vi "mMc emulator.vi"(2 "Command":string, 3 "error in (no error)":errorcluster) -> (7 "Return":string, 9 "error out":errorcluster)   [LabVIEW 2013]
uses:
  mMc param - global.vi
panel:
  out "Querry?":bool
  out "Param nn":dbl format="%.2f"
  out "Cmd":string
  out "Param xx":string
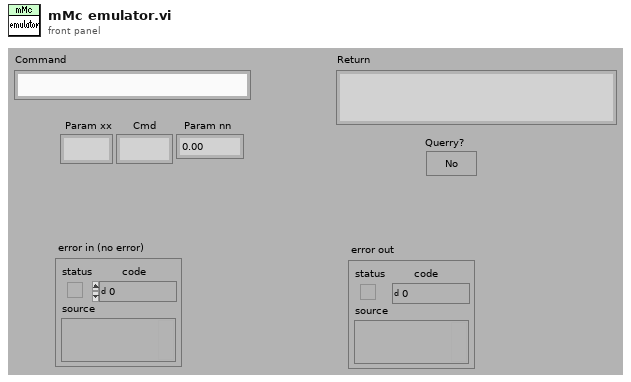
[diagram p1: front panel]
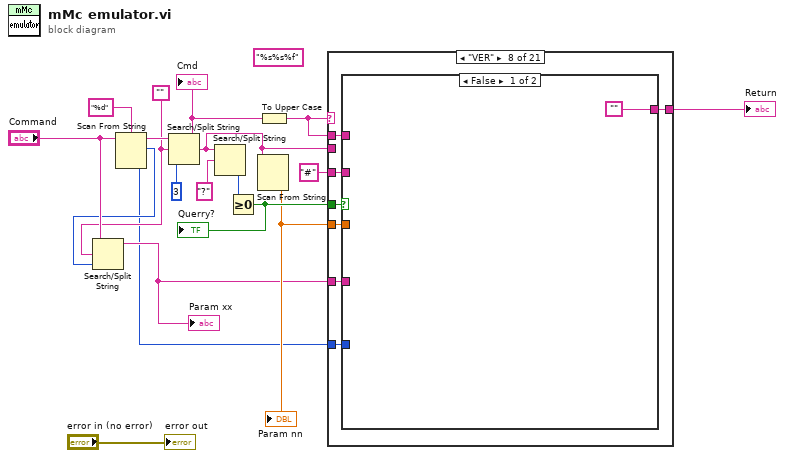
[diagram p0: block diagram]
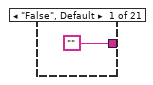
[diagram p2: hidden frame]
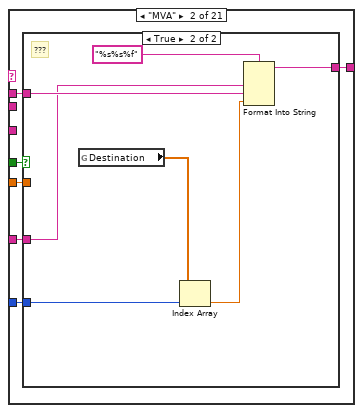
[diagram p3: hidden frame]
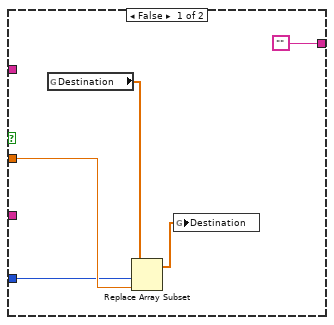
[diagram p4: hidden frame]
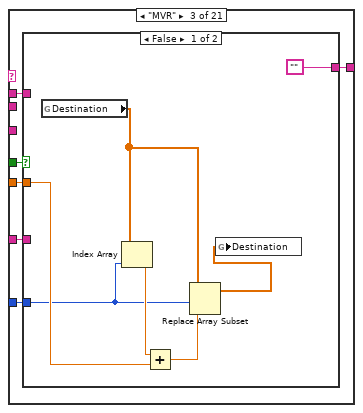
[diagram p5: hidden frame]
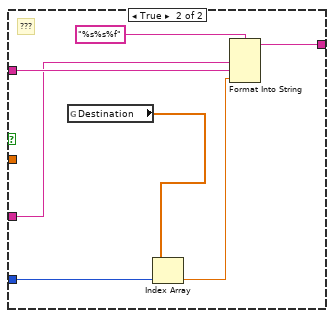
[diagram p6: hidden frame]
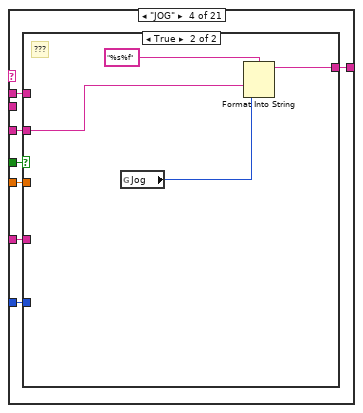
[diagram p7: hidden frame]
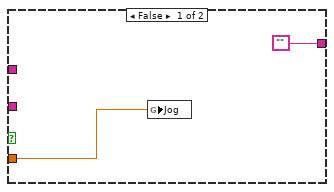
[diagram p8: hidden frame]
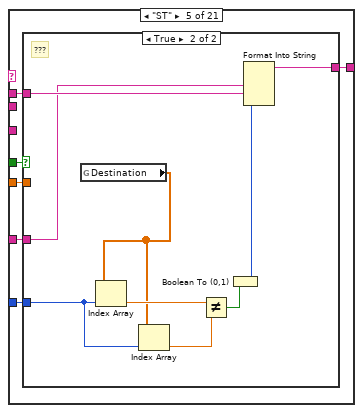
[diagram p9: hidden frame]
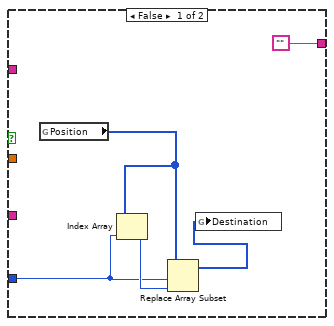
[diagram p10: hidden frame]
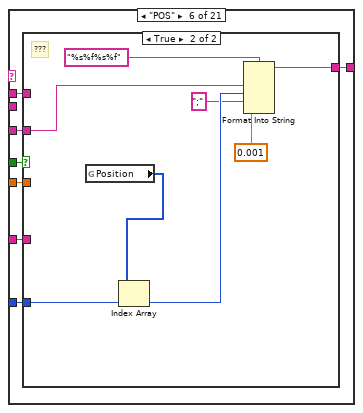
[diagram p11: hidden frame]
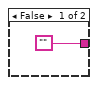
[diagram p12: hidden frame]
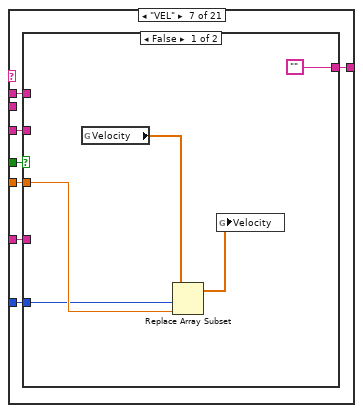
[diagram p13: hidden frame]
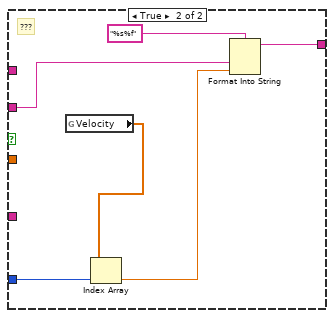
[diagram p14: hidden frame]
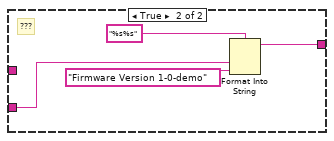
[diagram p15: hidden frame]
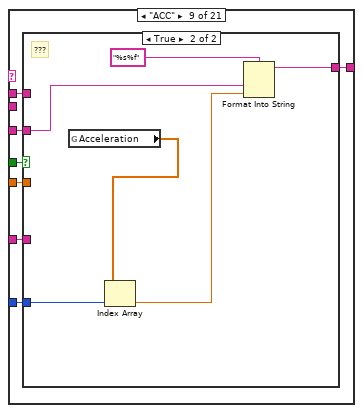
[diagram p16: hidden frame]
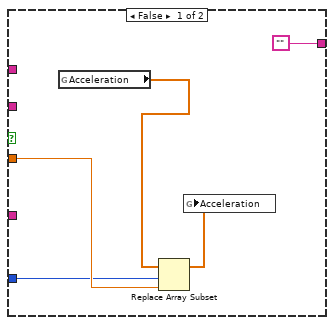
[diagram p17: hidden frame]
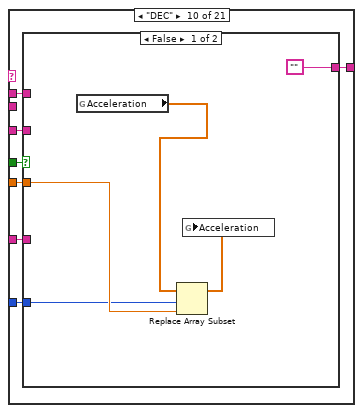
[diagram p18: hidden frame]
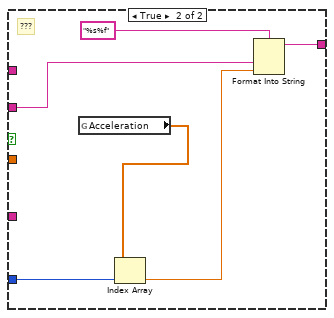
[diagram p19: hidden frame]
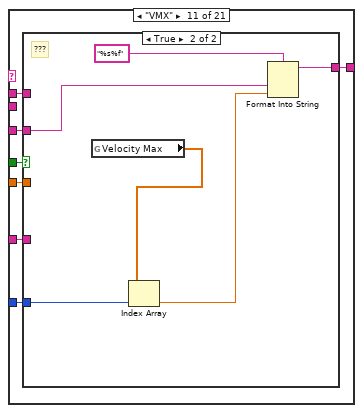
[diagram p20: hidden frame]
diagram:
  (unwired) "%s%s%f" ("Format String")
  w11 = ""
  n1 = Scan From String(format string="%d" ("Format String"), input string="Command") -> (remaining string=w18:string, offset past scan=w5:u32, output 1=w4:i32)  [unwired: 3 in, 1 out]
  n2 = Search/Split String(string="Command", search string/char (-)=w11, offset (0)=w5) -> (substring before match=w7:string)  [unwired: 2 out]
  "Param xx" <- w7
  n3 = Search/Split String(string=w18, search string/char (-)=w11, offset (0)=3) -> (substring before match=w14:string, match + rest of string=w2:string)  [unwired: 1 out]
  "Cmd" <- w14
  n4 = Search/Split String(string=w2, search string/char (-)="?") -> (offset of match=w15:i32)  [unwired: 1 in, 2 out]
  n5 = Greater Or Equal To 0?(x=w15) -> (x >= 0?=w13:bool)
  "Querry?" <- w13
  n6 = Scan From String(input string=w2) -> (output 1=w8:dbl)  [unwired: 4 in, 3 out]
  "Param nn" <- w8
  n7 = To Upper Case(1:w14) -> (0:w10:string)
  n8 = case shown="\"VER\"" w10 {
    tunnel: w13 -> [_ w25 w43 w64 w76 w97 w113 w131 w143 w161 w179 w197 w215 w233 w251 w269 w287 w305 w324 w342 w362]
    tunnel: w4 -> [_ w24 w42 w63 w75 w96 w112 w130 w142 w160 w178 w196 w214 w232 w250 w268 w286 w304 w323 w341 w361]
    tunnel: w7 -> [_ w22 w40 w61 w73 w94 w110 w128 w140 w158 w176 w194 w212 w230 w248 w266 w284 w302 w321 w339 w359]
    tunnel: w10 -> [_ w23 w41 w62 w74 w95 w111 w129 w141 w159 w177 w195 w213 w231 w249 w267 w285 w303 w322 w340 w360]
    tunnel: ["" w21 w39 w60 w72 w93 w109 w127 w139 w157 w175 w193 w211 w229 w247 w265 w283 w301 w320 w338 w358] -> w9
    tunnel: w8 -> [_ w20 w38 w59 w71 w92 w108 w126 w138 w156 w174 w192 w210 w228 w246 w264 w282 w300 w319 w337 w357]
    tunnel: w2 -> [_ _ _ _ _ _ _ _ _ _ _ _ _ _ _ _ _ _ w317 _ w356]
    tunnel: "#" ("Format String") -> [_ _ _ w58 _ w91 w107 w125 w137 w155 w173 w191 w209 w227 w245 w263 w281 w299 w318 w336 _]
    frame "False", Default {
    }
    frame "MVA" {
      n9 = case shown="True" w25 {
        tunnel: w24 -> [w26 w31]
        tunnel: w23 -> [_ w37]
        tunnel: w22 -> [_ w35]
        tunnel: ["" w34] -> w21
        tunnel: w20 -> [w29 _]
        frame False {
          n10 = global read "mMc param - global.vi" "Destination"() -> (w28:dbl[])
          n11 = Replace Array Subset(array=w28, new element=w29, index=w26) -> (w27:dbl[])
          n12 = global write "mMc param - global.vi" "Destination"(w27) -> ()
        }
        frame True {
          # "???"
          n13 = global read "mMc param - global.vi" "Destination"() -> (w32:dbl[])
          n14 = Index Array(array=w32, index=w31) -> (element=w36:dbl)
          n15 = Format Into String(format string="%s%s%f" ("Format String"), w35, w37, w36) -> (resulting string=w34:string)  [unwired: 2 in, 1 out]
        }
      }
    }
    frame "MVR" {
      n16 = case shown="False" w43 {
        tunnel: w42 -> [w44 w51]
        tunnel: w41 -> [_ w57]
        tunnel: w40 -> [_ w55]
        tunnel: ["" w54] -> w39
        tunnel: w38 -> [w49 _]
        frame False {
          n17 = global read "mMc param - global.vi" "Destination"() -> (w46:dbl[])
          n18 = Index Array(array=w46, index=w44) -> (element=w48:dbl)
          n19 = Add(x=w48, y=w49) -> (x+y=w47:dbl)
          n20 = Replace Array Subset(array=w46, new element=w47, index=w44) -> (w45:dbl[])
          n21 = global write "mMc param - global.vi" "Destination"(w45) -> ()
        }
        frame True {
          # "???"
          n22 = global read "mMc param - global.vi" "Destination"() -> (w52:dbl[])
          n23 = Index Array(array=w52, index=w51) -> (element=w56:dbl)
          n24 = Format Into String(format string="%s%s%f" ("Format String"), w55, w57, w56) -> (resulting string=w54:string)  [unwired: 2 in, 1 out]
        }
      }
    }
    frame "JOG" {
      n25 = case shown="True" w64 {
        tunnel: w63 -> [_ _]
        tunnel: w62 -> [_ _]
        tunnel: w61 -> [_ _]
        tunnel: ["" w70] -> w60
        tunnel: w59 -> [w65 _]
        tunnel: w58 -> [_ w67]
        frame False {
          n26 = global write "mMc param - global.vi" "Jog"(w65) -> ()
        }
        frame True {
          # "???"
          n27 = global read "mMc param - global.vi" "Jog"() -> (w68:i32)
          n28 = Format Into String(format string="%s%f" ("Format String"), w67, w68) -> (resulting string=w70:string)  [unwired: 2 in, 1 out]
        }
      }
    }
    frame "ST" {
      n29 = case shown="True" w76 {
        tunnel: w75 -> [w77 w82]
        tunnel: w74 -> [_ w90]
        tunnel: w73 -> [_ w89]
        tunnel: ["" w88] -> w72
        tunnel: w71 -> [_ _]
        frame False {
          n30 = global read "mMc param - global.vi" "Position"() -> (w79:i32[])
          n31 = Index Array(array=w79, index=w77) -> (element=w80:i32)
          n32 = Replace Array Subset(array=w79, new element=w80, index=w77) -> (w78:i32[])
          n33 = global write "mMc param - global.vi" "Destination"(w78) -> ()
        }
        frame True {
          # "???"
          n34 = global read "mMc param - global.vi" "Destination"() -> (w83:dbl[])
          n35 = Index Array(array=w83, index=w82) -> (element=w87:dbl)
          n36 = Index Array(array=w83, index=w82) -> (element=w86:dbl)
          n37 = Not Equal?(x=w87, y=w86) -> (x != y?=w85:bool)
          n38 = Boolean To (0,1)(Boolean=w85) -> (0, 1=w84:i16)
          n39 = Format Into String(w89, w90, w84) -> (resulting string=w88:string)  [unwired: 3 in, 1 out]
        }
      }
    }
    frame "POS" {
      n40 = case shown="True" w97 {
        tunnel: w96 -> [_ w99]
        tunnel: w95 -> [_ _]
        tunnel: w94 -> [_ _]
        tunnel: ["" w106] -> w93
        tunnel: w92 -> [_ _]
        tunnel: w91 -> [_ w102]
        frame False {
        }
        frame True {
          # "???"
          n41 = global read "mMc param - global.vi" "Position"() -> (w103:i32[])
          n42 = Index Array(array=w103, index=w99) -> (element=w105:i32)
          n43 = Format Into String(format string="%s%f%s%f" ("Format String"), w102, w105, ";" ("input 3"), 0.001 ("input 4")) -> (resulting string=w106:string)  [unwired: 2 in, 1 out]
        }
      }
    }
    frame "VEL" {
      n44 = case shown="False" w113 {
        tunnel: w112 -> [w114 w119]
        tunnel: w111 -> [_ _]
        tunnel: w110 -> [_ _]
        tunnel: ["" w124] -> w109
        tunnel: w108 -> [w117 _]
        tunnel: w107 -> [_ w120]
        frame False {
          n45 = global read "mMc param - global.vi" "Velocity"() -> (w115:dbl[])
          n46 = Replace Array Subset(array=w115, new element=w117, index=w114) -> (w116:dbl[])
          n47 = global write "mMc param - global.vi" "Velocity"(w116) -> ()
        }
        frame True {
          # "???"
          n48 = global read "mMc param - global.vi" "Velocity"() -> (w121:dbl[])
          n49 = Index Array(array=w121, index=w119) -> (element=w123:dbl)
          n50 = Format Into String(format string="%s%f" ("Format String"), w120, w123) -> (resulting string=w124:string)  [unwired: 2 in, 1 out]
        }
      }
    }
    frame "VER" {
      n51 = case shown="False" w131 {
        tunnel: w130 -> [_ _]
        tunnel: w129 -> [_ _]
        tunnel: w128 -> [_ _]
        tunnel: ["" w136] -> w127
        tunnel: w126 -> [_ _]
        tunnel: w125 -> [_ w134]
        frame False {
        }
        frame True {
          # "???"
          n52 = Format Into String(format string="%s%s" ("Format String"), w134, "Firmware Version 1-0-demo" ("input 2")) -> (resulting string=w136:string)  [unwired: 2 in, 1 out]
        }
      }
    }
    frame "ACC" {
      n53 = case shown="True" w143 {
        tunnel: w142 -> [w144 w149]
        tunnel: w141 -> [_ _]
        tunnel: w140 -> [_ _]
        tunnel: ["" w154] -> w139
        tunnel: w138 -> [w147 _]
        tunnel: w137 -> [_ w150]
        frame False {
          n54 = global read "mMc param - global.vi" "Acceleration"() -> (w145:dbl[])
          n55 = Replace Array Subset(array=w145, new element=w147, index=w144) -> (w146:dbl[])
          n56 = global write "mMc param - global.vi" "Acceleration"(w146) -> ()
        }
        frame True {
          # "???"
          n57 = global read "mMc param - global.vi" "Acceleration"() -> (w151:dbl[])
          n58 = Index Array(array=w151, index=w149) -> (element=w153:dbl)
          n59 = Format Into String(format string="%s%f" ("Format String"), w150, w153) -> (resulting string=w154:string)  [unwired: 2 in, 1 out]
        }
      }
    }
    frame "DEC" {
      n60 = case shown="False" w161 {
        tunnel: w160 -> [w162 w167]
        tunnel: w159 -> [_ _]
        tunnel: w158 -> [_ _]
        tunnel: ["" w168] -> w157
        tunnel: w156 -> [w163 _]
        tunnel: w155 -> [_ w169]
        frame False {
          n61 = global read "mMc param - global.vi" "Acceleration"() -> (w164:dbl[])
          n62 = Replace Array Subset(array=w164, new element=w163, index=w162) -> (w165:dbl[])
          n63 = global write "mMc param - global.vi" "Acceleration"(w165) -> ()
        }
        frame True {
          # "???"
          n64 = global read "mMc param - global.vi" "Acceleration"() -> (w170:dbl[])
          n65 = Index Array(array=w170, index=w167) -> (element=w172:dbl)
          n66 = Format Into String(format string="%s%f" ("Format String"), w169, w172) -> (resulting string=w168:string)  [unwired: 2 in, 1 out]
        }
      }
    }
    frame "VMX" {
      n67 = case shown="True" w179 {
        tunnel: w178 -> [w180 w185]
        tunnel: w177 -> [_ _]
        tunnel: w176 -> [_ _]
        tunnel: ["" w186] -> w175
        tunnel: w174 -> [w181 _]
        tunnel: w173 -> [_ w187]
        frame False {
          n68 = global read "mMc param - global.vi" "Velocity Max"() -> (w182:dbl[])
          n69 = Replace Array Subset(array=w182, new element=w181, index=w180) -> (w183:dbl[])
          n70 = global write "mMc param - global.vi" "Velocity Max"(w183) -> ()
        }
        frame True {
          # "???"
          n71 = global read "mMc param - global.vi" "Velocity Max"() -> (w188:dbl[])
          n72 = Index Array(array=w188, index=w185) -> (element=w190:dbl)
          n73 = Format Into String(format string="%s%f" ("Format String"), w187, w190) -> (resulting string=w186:string)  [unwired: 2 in, 1 out]
        }
      }
    }
    frame "AMX" {
      n74 = case shown="False" w197 {
        tunnel: w196 -> [w198 w203]
        tunnel: w195 -> [_ _]
        tunnel: w194 -> [_ _]
        tunnel: ["" w204] -> w193
        tunnel: w192 -> [w199 _]
        tunnel: w191 -> [_ w205]
        frame False {
          n75 = global read "mMc param - global.vi" "Acceleration Max"() -> (w200:dbl[])
          n76 = Replace Array Subset(array=w200, new element=w199, index=w198) -> (w201:dbl[])
          n77 = global write "mMc param - global.vi" "Acceleration Max"(w201) -> ()
        }
        frame True {
          # "???"
          n78 = global read "mMc param - global.vi" "Acceleration Max"() -> (w206:dbl[])
          n79 = Index Array(array=w206, index=w203) -> (element=w208:dbl)
          n80 = Format Into String(format string="%s%f" ("Format String"), w205, w208) -> (resulting string=w204:string)  [unwired: 2 in, 1 out]
        }
      }
    }
    frame "TLN" {
      n81 = case shown="True" w215 {
        tunnel: w214 -> [w216 w221]
        tunnel: w213 -> [_ _]
        tunnel: w212 -> [_ _]
        tunnel: ["" w222] -> w211
        tunnel: w210 -> [w217 _]
        tunnel: w209 -> [_ w223]
        frame False {
          n82 = global read "mMc param - global.vi" "Limit -"() -> (w218:dbl[])
          n83 = Replace Array Subset(array=w218, new element=w217, index=w216) -> (w219:dbl[])
          n84 = global write "mMc param - global.vi" "Limit -"(w219) -> ()
        }
        frame True {
          # "???"
          n85 = global read "mMc param - global.vi" "Limit -"() -> (w224:dbl[])
          n86 = Index Array(array=w224, index=w221) -> (element=w226:dbl)
          n87 = Format Into String(format string="%s%f" ("Format String"), w223, w226) -> (resulting string=w222:string)  [unwired: 2 in, 1 out]
        }
      }
    }
    frame "TLP" {
      n88 = case shown="False" w233 {
        tunnel: w232 -> [w234 w239]
        tunnel: w231 -> [_ _]
        tunnel: w230 -> [_ _]
        tunnel: ["" w240] -> w229
        tunnel: w228 -> [w235 _]
        tunnel: w227 -> [_ w241]
        frame False {
          n89 = global read "mMc param - global.vi" "Limit +"() -> (w236:dbl[])
          n90 = Replace Array Subset(array=w236, new element=w235, index=w234) -> (w237:dbl[])
          n91 = global write "mMc param - global.vi" "Limit +"(w237) -> ()
        }
        frame True {
          # "???"
          n92 = global read "mMc param - global.vi" "Limit +"() -> (w242:dbl[])
          n93 = Index Array(array=w242, index=w239) -> (element=w244:dbl)
          n94 = Format Into String(format string="%s%f" ("Format String"), w241, w244) -> (resulting string=w240:string)  [unwired: 2 in, 1 out]
        }
      }
    }
    frame "REZ" {
      n95 = case shown="True" w251 {
        tunnel: w250 -> [w252 w257]
        tunnel: w249 -> [_ _]
        tunnel: w248 -> [_ _]
        tunnel: ["" w258] -> w247
        tunnel: w246 -> [w253 _]
        tunnel: w245 -> [_ w259]
        frame False {
          n96 = global read "mMc param - global.vi" "Step Rezol"() -> (w254:dbl[])
          n97 = Replace Array Subset(array=w254, new element=w253, index=w252) -> (w255:dbl[])
          n98 = global write "mMc param - global.vi" "Step Rezol"(w255) -> ()
        }
        frame True {
          # "???"
          n99 = global read "mMc param - global.vi" "Step Rezol"() -> (w260:dbl[])
          n100 = Index Array(array=w260, index=w257) -> (element=w262:dbl)
          n101 = Format Into String(format string="%s%f" ("Format String"), w259, w262) -> (resulting string=w258:string)  [unwired: 2 in, 1 out]
        }
      }
    }
    frame "ENC" {
      n102 = case shown="False" w269 {
        tunnel: w268 -> [w270 w275]
        tunnel: w267 -> [_ _]
        tunnel: w266 -> [_ _]
        tunnel: ["" w276] -> w265
        tunnel: w264 -> [w271 _]
        tunnel: w263 -> [_ w277]
        frame False {
          n103 = global read "mMc param - global.vi" "Enc Rezol"() -> (w272:dbl[])
          n104 = Replace Array Subset(array=w272, new element=w271, index=w270) -> (w273:dbl[])
          n105 = global write "mMc param - global.vi" "Enc Rezol"(w273) -> ()
        }
        frame True {
          # "???"
          n106 = global read "mMc param - global.vi" "Enc Rezol"() -> (w278:dbl[])
          n107 = Index Array(array=w278, index=w275) -> (element=w280:dbl)
          n108 = Format Into String(format string="%s%f" ("Format String"), w277, w280) -> (resulting string=w276:string)  [unwired: 2 in, 1 out]
        }
      }
    }
    frame "JAC" {
      n109 = case shown="False" w287 {
        tunnel: w286 -> [w288 w293]
        tunnel: w285 -> [_ _]
        tunnel: w284 -> [_ _]
        tunnel: ["" w294] -> w283
        tunnel: w282 -> [w289 _]
        tunnel: w281 -> [_ w295]
        frame False {
          n110 = global read "mMc param - global.vi" "Jog Acc"() -> (w290:dbl[])
          n111 = Replace Array Subset(array=w290, new element=w289, index=w288) -> (w291:dbl[])
          n112 = global write "mMc param - global.vi" "Jog Acc"(w291) -> ()
        }
        frame True {
          n113 = global read "mMc param - global.vi" "Jog Acc"() -> (w296:dbl[])
          n114 = Index Array(array=w296, index=w293) -> (element=w298:dbl)
          n115 = Format Into String(format string="%s%f" ("Format String"), w295, w298) -> (resulting string=w294:string)  [unwired: 2 in, 1 out]
        }
      }
    }
    frame "DBD" {
      n116 = case shown="True" w305 {
        tunnel: w304 -> [w306 w311]
        tunnel: w303 -> [_ _]
        tunnel: w302 -> [_ _]
        tunnel: ["" w312] -> w301
        tunnel: w300 -> [w307 _]
        tunnel: w299 -> [_ w313]
        frame False {
          n117 = global read "mMc param - global.vi" "deadband"() -> (w308:dbl[])
          n118 = Replace Array Subset(array=w308, new element=w307, index=w306) -> (w309:dbl[])
          n119 = global write "mMc param - global.vi" "deadband"(w309) -> ()
        }
        frame True {
          n120 = global read "mMc param - global.vi" "deadband"() -> (w314:dbl[])
          n121 = Index Array(array=w314, index=w311) -> (element=w316:dbl)
          n122 = Format Into String(format string="%s%f" ("Format String"), w313, w316) -> (resulting string=w312:string)  [unwired: 2 in, 1 out]
        }
      }
    }
    frame "PID" {
      n123 = case shown="True" w324 {
        tunnel: w323 -> [w326 w330]
        tunnel: w322 -> [_ _]
        tunnel: w321 -> [_ _]
        tunnel: ["" w331] -> w320
        tunnel: w319 -> [_ _]
        tunnel: w318 -> [_ w332]
        tunnel: w317 -> [w325 _]
        frame False {
          n124 = global read "mMc param - global.vi" "PID"() -> (w327:string[])
          n125 = Replace Array Subset(array=w327, new element=w325, index=w326) -> (w328:string[])
          n126 = global write "mMc param - global.vi" "PID"(w328) -> ()
        }
        frame True {
          n127 = global read "mMc param - global.vi" "PID"() -> (w333:string[])
          n128 = Index Array(array=w333, index=w330) -> (element=w335:string)
          n129 = Format Into String(format string="%s%s" ("Format String"), w332, w335) -> (resulting string=w331:string)  [unwired: 2 in, 1 out]
        }
      }
    }
    frame "FBK" {
      n130 = case shown="False" w342 {
        tunnel: w341 -> [w344 w350]
        tunnel: w340 -> [_ _]
        tunnel: w339 -> [_ _]
        tunnel: ["" w351] -> w338
        tunnel: w337 -> [w345 _]
        tunnel: w336 -> [_ w352]
        frame False {
          n131 = Greater Than 0?(x=w345) -> (x > 0?=w343:bool)
          n132 = global read "mMc param - global.vi" "feedback"() -> (w346:bool[])
          n133 = Replace Array Subset(array=w346, new element=w343, index=w344) -> (w347:bool[])
          n134 = global write "mMc param - global.vi" "feedback"(w347) -> ()
        }
        frame True {
          n135 = global read "mMc param - global.vi" "feedback"() -> (w353:bool[])
          n136 = Index Array(array=w353, index=w350) -> (element=w355:bool)
          n137 = Boolean To (0,1)(Boolean=w355) -> (0, 1=w349:i16)
          n138 = Format Into String(format string="%s%d" ("Format String"), w352, w349) -> (resulting string=w351:string)  [unwired: 2 in, 1 out]
        }
      }
    }
    frame "STP" {
      n139 = case shown="True" w362 {
        tunnel: w361 -> [_ _]
        tunnel: w360 -> [_ _]
        tunnel: w359 -> [_ _]
        tunnel: ["" ""] -> w358
        tunnel: w357 -> [_ _]
        tunnel: w356 -> [_ _]
        frame False {
        }
        frame True {
          # "???"
        }
      }
    }
  }
  "Return" <- w9
  "error out" <- "error in (no error)"
